vi "XML.Limits.Generate.vi"(8 "error in":errorcluster, 9 "Root name":string="LimitFile", 10 "seqs in":T1[](array[typedef]), 11 "XML file path":path) -> (0 "error out":errorcluster)   [LabVIEW 2019, in "Tools.lvlib"]
uses:
  Tools.lvlib
  LibXML/LibXML.lvlib
  TestStand/Export limits/controls/TS.Seq.Step.Type.ctl
  TestStand/Export limits/controls/TS.Seq.Type.ctl
panel:
  out "Limits":string[][](array[string])
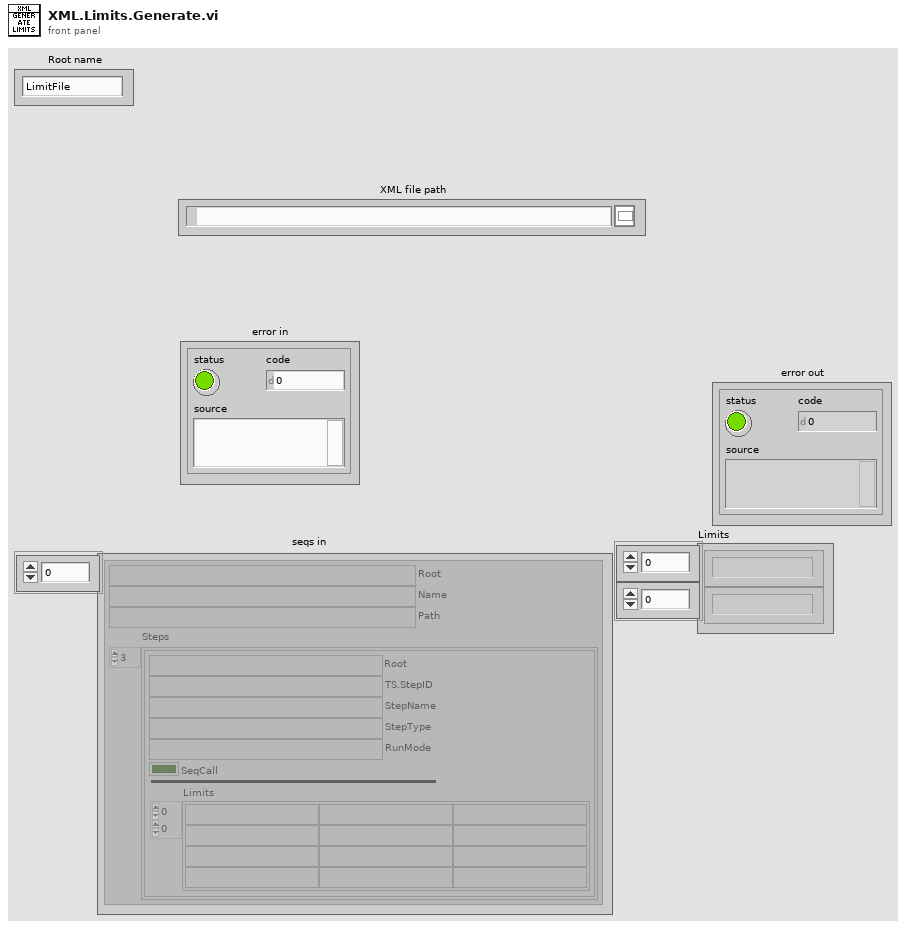
[diagram p1: front panel]
types:
  T1 = typedef "TS.Seq.Type.ctl" = cluster{"Root":string, "Name":string, "Path":string, "Steps":T2[]}
  T2 = typedef "TS.Seq.Step.Type.ctl" = cluster{"Root":string, "TS.StepID":string, "StepName":string, "StepType":string, "RunMode":string, "SeqCall":bool, "Limits":string[][]}
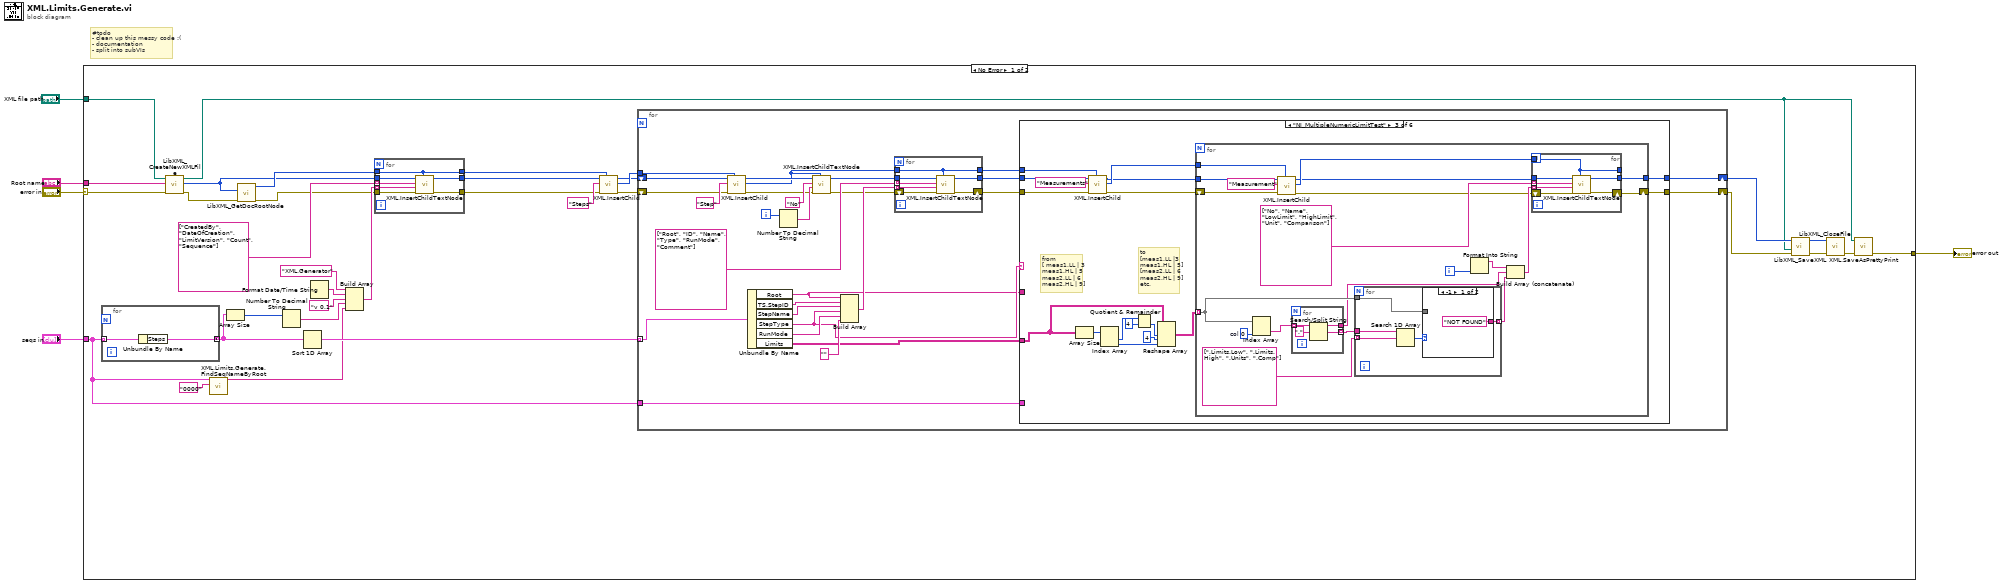
[diagram p0: block diagram]
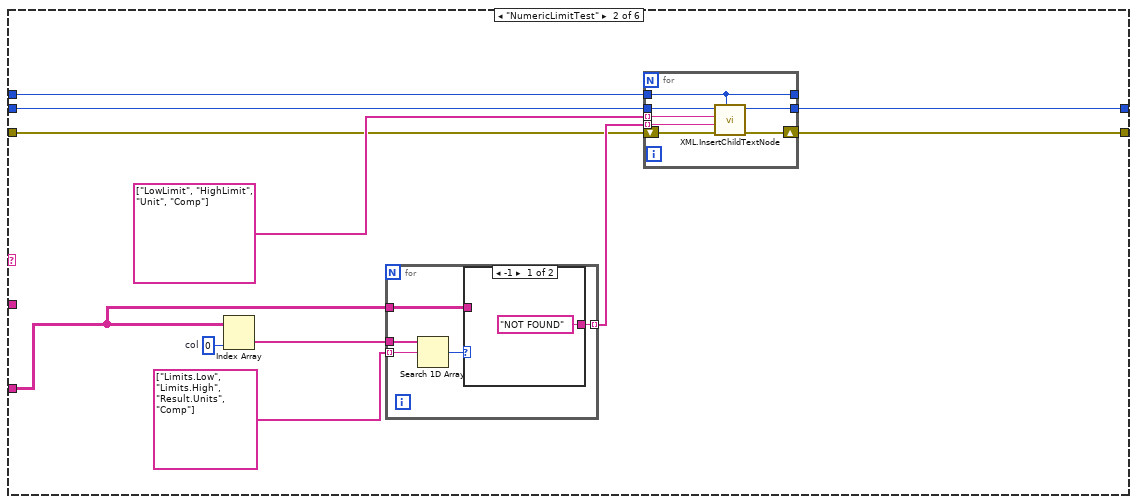
[diagram p3: hidden frame]
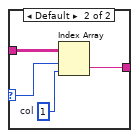
[diagram p4: hidden frame]
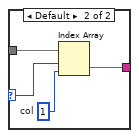
[diagram p5: hidden frame]
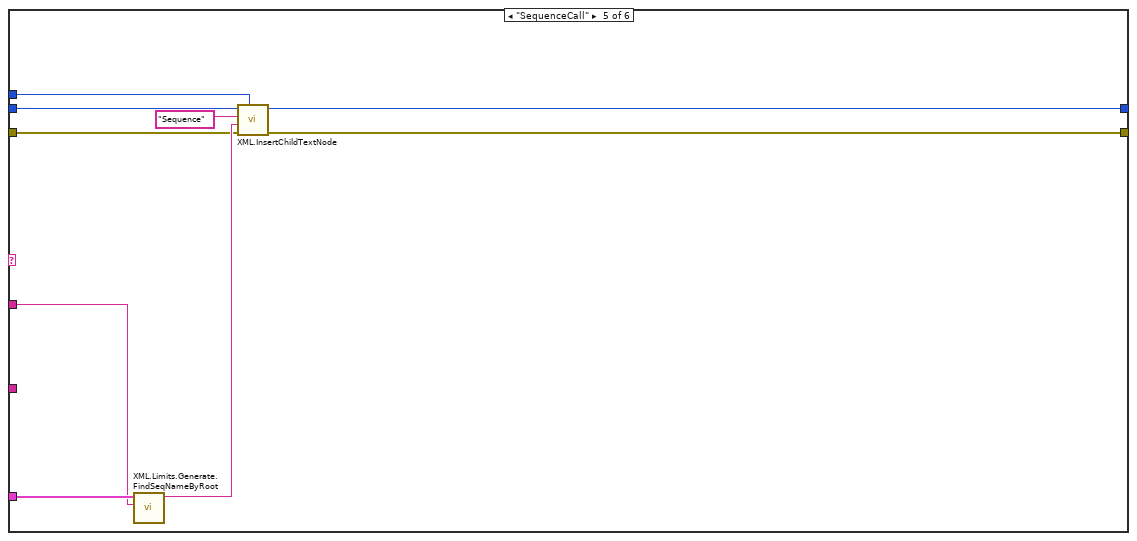
[diagram p7: hidden frame]
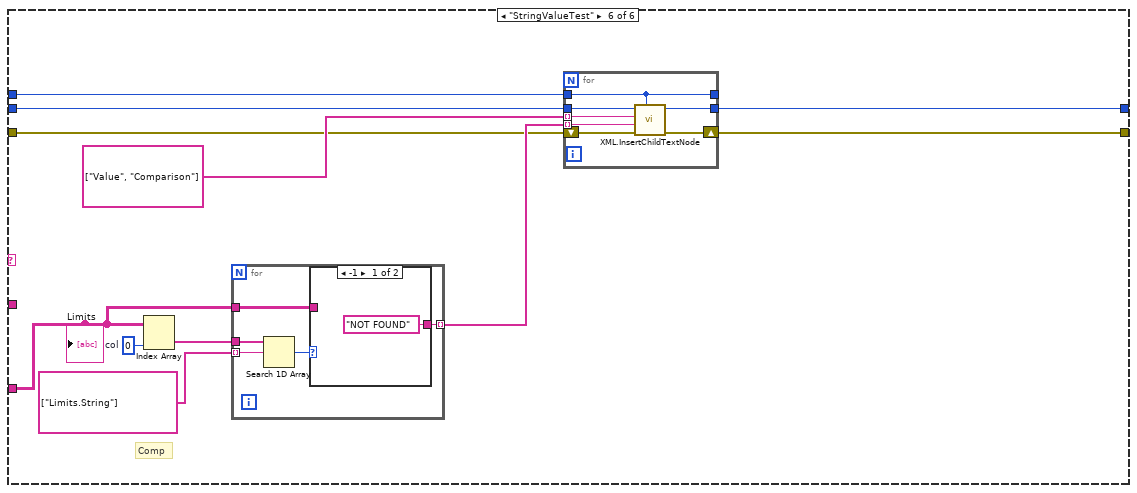
[diagram p8: hidden frame]
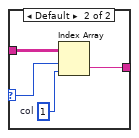
[diagram p9: hidden frame]
diagram:
  # "#todo \n- clean up this messy code :(\n- documentation\n- split into subVIs"
  n1 = case shown="No Error" "error in" {
    selector: "error in" -> [w18 w210]
    tunnel: "seqs in" -> [w22 _]
    tunnel: [w8 w210] -> w3
    tunnel: "Root name" -> [w19 _]
    tunnel: "XML file path" -> [w7 _]
    frame No Error {
      n2 = for {
        tunnel: w22 -> [w202] mode=indexing
        tunnel: [w201] -> w26 mode=concatenating
        n3 = Unbundle By Name(w202) -> ("Steps"=w201:T2[])
      }
      n4 = call "LibXML_CreateNewXMLFile.vi"("error in"=w18, "Root element name"=w19, "file path"=w7) -> ("error out"=w15:errorcluster, "new doc out"=w14:u32, "new file path"=w6:path)  [unwired: 6 in]
      n5 = call "XML.Limits.Generate.FindSeqNameByRoot.vi"("root"="0000" ("y"), "seqs in"=w22) -> ("sequence"=w23:string)  [unwired: 9 in]
      n6 = Array Size(array=w26) -> (size(s)=w33:i32)
      n7 = call "LibXML_GetDocRootNode.vi"("error in"=w15, "doc"=w14) -> ("error out"=w17:errorcluster, "root node out"=w16:u32)  [unwired: 8 in]
      n8 = Number To Decimal String(number=w33) -> (decimal integer string=w32:string)  [unwired: 1 in]
      n9 = Sort 1D Array(array=w26) -> (sorted array=w25:T2[])
      n10 = Format Date/Time String() -> (date/time string=w35:string)  [unwired: 3 in]
      n11 = Build Array("XML.Generator" ("Tag Name"), w35, "v 0.1" ("element"), w32, w23) -> (w36:string[])
      n12 = for {
        tunnel: string[] ["CreatedBy", "DateOfCreation", "LimitVersion", "Count", "Sequence"] -> [w209] mode=indexing
        tunnel: w14 -> [w206]
        tunnel: w16 -> [w205]
        tunnel: w36 -> [w208] mode=indexing
        tunnel: [w207] -> w29
        tunnel: [w205] -> w27
        tunnel: w17 -> [w204]
        tunnel: [w203] -> w21
        n13 = call "XML.InsertChildTextNode.vi"("parent"=w205, "error in"=w204, "text"=w208, "name"=w209, "doc"=w206) -> ("error out"=w203:errorcluster, "doc out"=w207:u32)  [unwired: 5 in]
      }
      n14 = call "XML.InsertChild.vi"("parent"=w27, "error in"=w21, "name"="Steps" ("Tag Name"), "doc"=w29) -> ("error out"=w20:errorcluster, "new node"=w31:u32, "doc out"=w28:u32)  [unwired: 5 in]
      n15 = for {
        tunnel: w25 -> [w54] mode=indexing
        tunnel: w31 -> [w65]
        shift-right: [w63] -> w9
        shift-left: w28 -> [w64]
        tunnel: w22 -> [w45]
        shift-right: [w39] -> w11
        shift-left: w20 -> [w43]
        i -> [w66]
        n16 = call "XML.InsertChild.vi"("parent"=w65, "error in"=w43, "name"="Step" ("Tag Name"), "doc"=w64) -> ("error out"=w42:errorcluster, "new node"=w57:u32, "doc out"=w59:u32)  [unwired: 5 in]
        n17 = Unbundle By Name(w54) -> ("Root"=w44:string, "TS.StepID"=w53:string, "StepName"=w52:string, "StepType"=w48:string, "RunMode"=w51:string, "Limits"=w46:string[][])
        n18 = Number To Decimal String(number=w66) -> (decimal integer string=w61:string)  [unwired: 1 in]
        n19 = call "XML.InsertChildTextNode.vi"("parent"=w57, "error in"=w42, "text"=w61, "name"="No" ("Tag Name"), "doc"=w59) -> ("error out"=w41:errorcluster, "doc out"=w58:u32)  [unwired: 5 in]
        n20 = Build Array(w44, w53, w52, w48, w51, "" ("element")) -> (w49:string[])
        n21 = for {
          tunnel: [w200] -> w47
          tunnel: w58 -> [w199]
          tunnel: w57 -> [w198]
          tunnel: [w198] -> w56
          tunnel: string[] ["Root", "ID", "Name", "Type", "RunMode", "Comment"] -> [w197] mode=indexing
          tunnel: w49 -> [w196] mode=indexing
          shift-right: [w194] -> w40
          shift-left: w41 -> [w195]
          n22 = call "XML.InsertChildTextNode.vi"("parent"=w198, "error in"=w195, "text"=w196, "name"=w197, "doc"=w199) -> ("error out"=w194:errorcluster, "doc out"=w200:u32)  [unwired: 5 in]
        }
        n23 = case shown="\"NI_MultipleNumericLimitTest\"" w48 {
          tunnel: [w68 w71 w113 w156 w163 w168] -> w63
          tunnel: w56 -> [_ w74 w112 _ w164 w176]
          tunnel: w47 -> [w68 w73 w111 w156 w165 w175]
          tunnel: w46 -> [_ w72 w101 _ _ w170]
          tunnel: w45 -> [_ _ _ _ w160 _]
          tunnel: w44 -> [_ _ _ _ w159 _]
          tunnel: w40 -> [w67 w70 w99 w155 w158 w167]
          tunnel: [w67 w69 w97 w155 w157 w166] -> w39
          frame "PassFailTest" {
          }
          frame "NumericLimitTest" {
            w78 = 0  # col
            n24 = Index Array(array=w72, index (col)=w78) -> (element=w77:string[])  [unwired: 1 in]
            n25 = for {
              tunnel: w77 -> [w84]
              tunnel: string[] ["Limits.Low", "Limits.High", "Result.Units", "Comp"] -> [w83] mode=indexing
              tunnel: w72 -> [w81]
              tunnel: [w80] -> w75 mode=indexing
              n26 = Search 1D Array(1D array=w84, element=w83) -> (index of element=w82:i32)  [unwired: 1 in]
              n27 = case shown="-1" w82 {
                selector: w82 -> [_ w87]
                tunnel: w81 -> [_ w88]
                tunnel: ["NOT FOUND" ("String") w86] -> w80
                frame -1 {
                }
                frame Default {
                  w89 = 1  # col
                  n28 = Index Array(array=w88, index (row)=w87, index (col)=w89) -> (element=w86:string)
                }
              }
            }
            n29 = for {
              tunnel: [w96] -> w71
              tunnel: w73 -> [w95]
              tunnel: w74 -> [w94]
              tunnel: [w94] -> _
              tunnel: string[] ["LowLimit", "HighLimit", "Unit", "Comp"] -> [w93] mode=indexing
              tunnel: w75 -> [w92] mode=indexing
              shift-right: [w90] -> w69
              shift-left: w70 -> [w91]
              n30 = call "XML.InsertChildTextNode.vi"("parent"=w94, "error in"=w91, "text"=w92, "name"=w93, "doc"=w95) -> ("error out"=w90:errorcluster, "doc out"=w96:u32)  [unwired: 5 in]
            }
          }
          frame "NI_MultipleNumericLimitTest" {
            # "to\n[meas1.LL |3 \nmeas1.HL | 5]\n[meas2.LL | 6\nmeas2.HL | 9]\netc."
            # "from \n[ meas1.LL | 3\nmeas1.HL | 5\nmeas2.LL | 6\nmeas2.HL | 9]"
            n31 = Array Size(array=w101) -> (size(s)=w102:i32[])
            n32 = call "XML.InsertChild.vi"("parent"=w112, "error in"=w99, "name"="Measurements", "doc"=w111) -> ("error out"=w98:errorcluster, "new node"=w109:u32, "doc out"=w108:u32)  [unwired: 5 in]
            n33 = Index Array(array=w102) -> (element #1=w103:i32, element #2=w107:i32)  [unwired: 2 in]
            n34 = Quotient & Remainder(x=w103, y=4) -> (floor(x/y)=w105:i32)  [unwired: 1 out]
            n35 = Reshape Array(w101, w105, 4 ("dimension size"), w107) -> (w100:string[][][])
            n36 = for {
              tunnel: [w130] -> w113
              tunnel: w100 -> [w129] mode=indexing
              tunnel: w109 -> [w127]
              tunnel: w108 -> [w125]
              shift-right: [w114] -> w97
              shift-left: w98 -> [w116]
              i -> [w121]
              w132 = 0  # col
              n37 = Index Array(array=w129, index (col)=w132) -> (element=w119:string[])  [unwired: 1 in]
              n38 = call "XML.InsertChild.vi"("parent"=w127, "error in"=w116, "name"="Measurement", "doc"=w125) -> ("error out"=w115:errorcluster, "new node"=w126:u32, "doc out"=w124:u32)  [unwired: 5 in]
              n39 = for {
                tunnel: w119 -> [w137] mode=indexing
                tunnel: [w135] -> w118
                tunnel: [w134] -> w117 mode=indexing
                n40 = Search/Split String(string=w137, search string/char (-)=".") -> (substring before match=w135:string, match + rest of string=w134:string)  [unwired: 1 in, 1 out]
              }
              n41 = for {
                tunnel: w117 -> [w142]
                tunnel: string[] [".Limits.Low", ".Limits.High", ".Units", ".Comp"] -> [w141] mode=indexing
                tunnel: w129 -> [w139]
                tunnel: [w138] -> w122 mode=indexing
                n42 = Search 1D Array(1D array=w142, element=w141) -> (index of element=w140:i32)  [unwired: 1 in]
                n43 = case shown="-1" w140 {
                  selector: w140 -> [_ w145]
                  tunnel: w139 -> [_ w146]
                  tunnel: ["NOT FOUND" ("String") w144] -> w138
                  frame -1 {
                  }
                  frame Default {
                    w147 = 1  # col
                    n44 = Index Array(array=w146, index (row)=w145, index (col)=w147) -> (element=w144:string)
                  }
                }
              }
              n45 = Format Into String(w121) -> (resulting string=w120:string)  [unwired: 3 in, 1 out]
              n46 = Build Array (concatenate)(w120, w118, w122) -> (w123:string[])
              n47 = for {
                tunnel: [w154] -> w130
                tunnel: w124 -> [w153]
                tunnel: w126 -> [w152]
                tunnel: [w152] -> _
                tunnel: string[] ["No", "Name", "LowLimit", "HighLimit", "Unit", "Comparison"] -> [w151] mode=indexing
                tunnel: w123 -> [w150] mode=indexing
                shift-right: [w148] -> w114
                shift-left: w115 -> [w149]
                n48 = call "XML.InsertChildTextNode.vi"("parent"=w152, "error in"=w149, "text"=w150, "name"=w151, "doc"=w153) -> ("error out"=w148:errorcluster, "doc out"=w154:u32)  [unwired: 5 in]
              }
            }
          }
          frame Default {
          }
          frame "SequenceCall" {
            n49 = call "XML.Limits.Generate.FindSeqNameByRoot.vi"("root"=w159, "seqs in"=w160) -> ("sequence"=w161:string)  [unwired: 9 in]
            n50 = call "XML.InsertChildTextNode.vi"("parent"=w164, "error in"=w158, "text"=w161, "name"="Sequence", "doc"=w165) -> ("error out"=w157:errorcluster, "doc out"=w163:u32)  [unwired: 5 in]
          }
          frame "StringValueTest" {
            w173 = 0  # col
            # "Comp"
            n51 = Index Array(array=w170, index (col)=w173) -> (element=w172:string[])  [unwired: 1 in]
            n52 = for {
              tunnel: w172 -> [w181]
              tunnel: string[] ["Limits.String"] -> [w180] mode=indexing
              tunnel: w170 -> [w178]
              tunnel: [w177] -> w169 mode=indexing
              n53 = Search 1D Array(1D array=w181, element=w180) -> (index of element=w179:i32)  [unwired: 1 in]
              n54 = case shown="-1" w179 {
                selector: w179 -> [_ w184]
                tunnel: w178 -> [_ w185]
                tunnel: ["NOT FOUND" ("String") w183] -> w177
                frame -1 {
                }
                frame Default {
                  w186 = 1  # col
                  n55 = Index Array(array=w185, index (row)=w184, index (col)=w186) -> (element=w183:string)
                }
              }
            }
            n56 = for {
              tunnel: [w193] -> w168
              tunnel: w175 -> [w192]
              tunnel: w176 -> [w191]
              tunnel: [w191] -> _
              tunnel: string[] ["Value", "Comparison"] -> [w190] mode=indexing
              tunnel: w169 -> [w189] mode=indexing
              shift-right: [w187] -> w166
              shift-left: w167 -> [w188]
              n57 = call "XML.InsertChildTextNode.vi"("parent"=w191, "error in"=w188, "text"=w189, "name"=w190, "doc"=w192) -> ("error out"=w187:errorcluster, "doc out"=w193:u32)  [unwired: 5 in]
            }
            "Limits" <- w170
          }
        }
      }
      n58 = call "LibXML_SaveXML.vi"("error in"=w11, "file path (dialog if empty)"=w6, "doc"=w9) -> ("error out"=w10:errorcluster, "doc copy out"=w13:u32)  [unwired: 6 in, 1 out]
      n59 = call "LibXML_CloseFile.vi"("error in"=w10, "doc"=w13) -> ("error out"=w12:errorcluster)  [unwired: 9 in]
      n60 = call "XML.SaveAsPrettyPrint.vi"("error in (no error)"=w12, "XML file path"=w6) -> ("error out"=w8:errorcluster)  [unwired: 9 in]
    }
    frame Error {
    }
  }
  "error out" <- w3
